vi "TextLog-Quit Log.vi"(11 "error in":errorcluster) -> (15 "error out":errorcluster)   [LabVIEW 2020]
uses:
  TextLog-Queue Data.ctl
  TextLog-Command.ctl
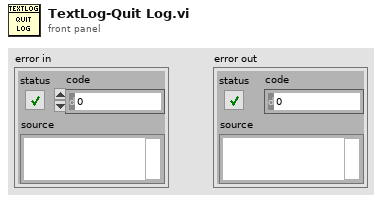
[diagram p1: front panel]
types:
  T1 = typedef "TextLog-Command.ctl" = enum16{"Unspecified", "Start", "Stop", "Quit", "Rename", "Make entry"}
  T2 = typedef "TextLog-Queue Data.ctl" = cluster{"Time":string, "Command":T1, "Message":string, "Data":string}
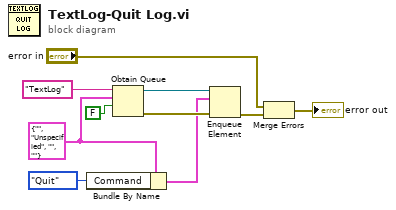
[diagram p0: block diagram]
diagram:
  w8 = T2 {"Time"="", "Command"=enum."Unspecified", "Message"="", "Data"=""} ("Trace Data")
  n1 = Bundle By Name(cluster=w8, "Command"=TextLog-Command."Quit") -> (w5:T2)
  n2 = Obtain Queue(name (unnamed)="TextLog", element data type=w8, create if not found? (T)=FALSE) -> (queue out=w7:refnum<queue>, error out=w6:errorcluster)  [unwired: 2 in, 1 out]
  n3 = Enqueue Element(queue=w7, element=w5, error in (no error)=w6) -> (error out=w4:errorcluster)  [unwired: 1 in, 2 out]
  n4 = Merge Errors("error in", w4) -> (→"error out":errorcluster)
